vi "Set example module data API.vi"(7 "Config":T1={"Type"=enum."PTI", "Wavelength (nm)"=600.0, "Wavelength (nm)"="600 nm", "Grating, gr/mm"=2, "Grating mode"=enum."Unknown", "Spectrum mode"={"Spectrum mode?"=FALSE, "Start wavelength (nm)"=0.0, "End wavelength (nm)"=0.0, "Wavelength step (nm)"=0.0, "Wavelength array"=[], "array index"=0}, "VISA"={"delay before read (ms)"=50, "Mono 1"={"Timeout (ms)"=1000, "Resource Name"="COM1", "Baud Rate"=9600, "Data Bits"=8, "Parity"=0, "Stop Bits"=10, "Flow Control"=0}, "Mono 2"={"Timeout (ms)"=1000, "Resource Name"="COM1", "Baud Rate"=9600, "Data Bits"=8, "Parity"=0, "Stop Bits"=10, "Flow Control"=0}}} {"VISA"."Mono 2"."Flow Control" items=["1.0"=10, "1.5"=15, "2.0"=20]; "VISA"."Mono 2"."Stop Bits" items=["None", "Odd", "Even", "Mark", "Space"]; "VISA"."Mono 2"."Parity" items=["None", "Odd", "Even", "Mark", "Space"]; "VISA"."Mono 1"."Flow Control" items=["1.0"=10, "1.5"=15, "2.0"=20]; "VISA"."Mono 1"."Stop Bits" items=["None", "Odd", "Even", "Mark", "Space"]; "VISA"."Mono 1"."Parity" items=["None", "Odd", "Even", "Mark", "Space"]; "Grating, gr/mm" items=["2400", "1800", "1200", "600", "300", "150"]}, 8 "Error In":errorcluster) -> (0 "Error Out":errorcluster)   [LabVIEW 2017, in "Main controller.lvlib"]
uses:
  Main controller.lvlib
  Example Module/Controls/Params.ctl
  Monochromator/Controls/Grating.ctl
  Monochromator/Controls/VISA parameters.ctl
  CTLs/Command Data [cluster].ctl
  CTLs/Commands [enum].ctl
  Events/Events.lvlib
  Serial comms/Serial comms.lvlib
  Monochromator/Monochromator.lvlib
  Example Module/Example Module.lvlib
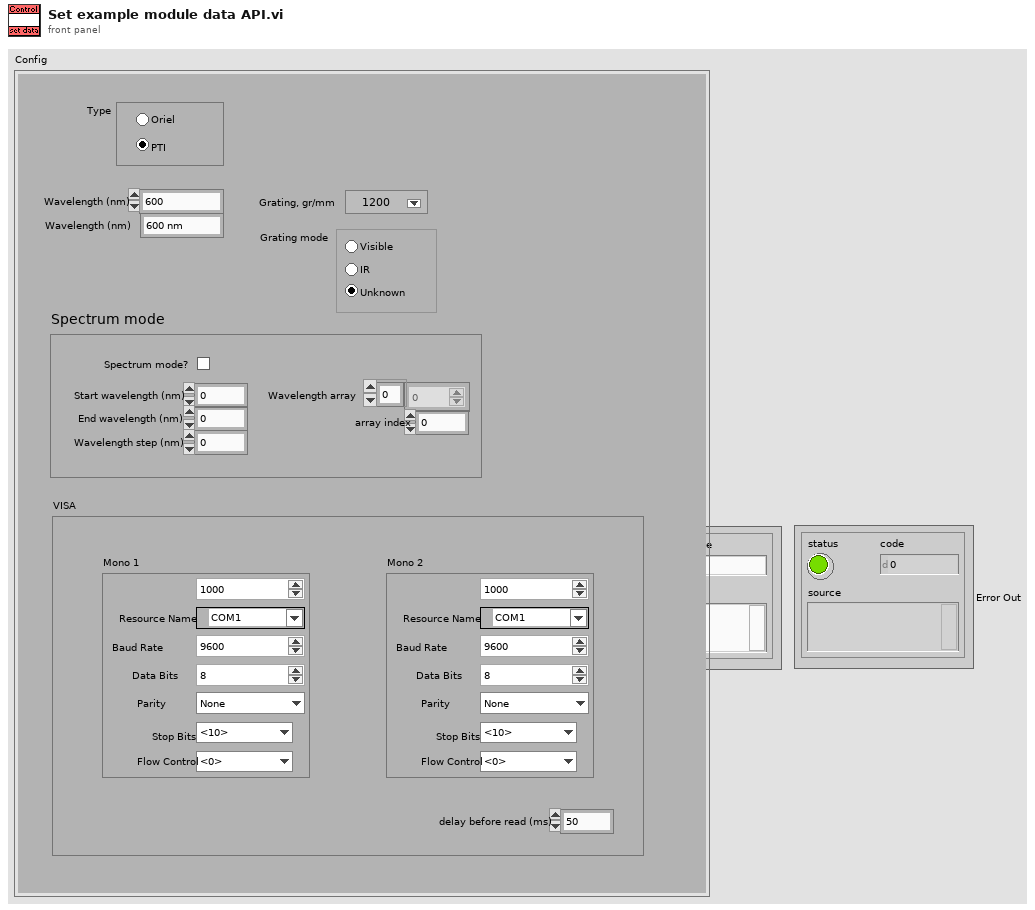
[diagram p1: front panel]
types:
  T1 = typedef "Example Module.lvlib/Params.ctl" = cluster{"Type":enum32{"Oriel", "PTI"}, "Wavelength (nm)":dbl, "Wavelength (nm)":string, "Grating, gr/mm":u16, "Grating mode":T2, "Spectrum mode":cluster{"Spectrum mode?":bool, "Start wavelength (nm)":dbl, "End wavelength (nm)":dbl, "Wavelength step (nm)":dbl, "Wavelength array":dbl[], "array index":u32}, "VISA":cluster{"delay before read (ms)":u32, "Mono 1":T3, "Mono 2":T3}}
  T2 = typedef "Monochromator.lvlib/Grating.ctl" = enum32{"Unknown", "Visible", "IR"}
  T3 = typedef "Serial comms.lvlib/VISA parameters.ctl" = cluster{"Timeout (ms)":u32, "Resource Name":refnum<visa-resource-name>, "Baud Rate":u32, "Data Bits":u16, "Parity":u16, "Stop Bits":u16, "Flow Control":u16}
  T4 = typedef "Main controller.lvlib/Command Data [cluster].ctl" = cluster{"Command":T5, "Data":variant}
  T5 = typedef "Main controller.lvlib/Commands [enum].ctl" = enum16{"Start", "Initialise Devices", "Stop", "Set DAQ data", "Set Scope data", "Set Spectrum Setup", "Spectrum Setup Complete", "Set Monochromator Setup", "Monochromator Setup Complete", "Set Monochromator data", "Set Colour Wheel Setup", "Colour Wheel Setup Complete", "Move Shutter", "Move Shutter Complete", "Collect Data", "DAQ Acquisition Complete", "Scope Acquisition Complete", "Collect Data Complete", "A-B Processing", "A-B Processing Complete", "DAQ-Scope Stitching", "DAQ-Scope Stitching Complete", "Return Shutter", "Return Shutter Complete", "Set colour wheel data", "Set all config data", "Acquire test data", "Accumulate test data", "Average test data", "All Averaging Complete", "DAQ Averaging Complete", "Scope Averaging Complete", "Finalise test data", "All Finalising Complete", "DAQ Finalising Complete", "Scope Finalising Complete", "Process test data", "End Test"}
  T6 = typedef "Events.lvlib/Refs [cluster].ctl" = cluster{"Exit":refnum<user-event>, "Controller":refnum<user-event>, "System Error":refnum<user-event>, "UI":refnum<user-event>, "Example Module":refnum<user-event>, "Shutter":refnum<user-event>, "Monochromator":refnum<user-event>, "DAQ":refnum<user-event>, "Scope":refnum<user-event>, "Processing":refnum<user-event>, "File IO":refnum<user-event>, "Colour wheel":refnum<user-event>}
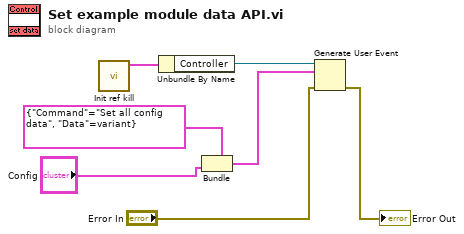
[diagram p0: block diagram]
diagram:
  n1 = call "Init ref kill.vi"() -> ("Messages"=w7:T6)  [unwired: 10 in, 1 out]
  n2 = Unbundle By Name(w7) -> ("Controller"=w6:refnum<user-event>)
  n3 = Bundle(cluster=T4 {"Command"=enum."Set all config data", "Data"=variant} ("event data"), "Data"="Config") -> (w2:T4)  [unwired: 1 in]
  n4 = Generate User Event(user event=w6, event data cluster=w2, error in="Error In") -> (error out=→"Error Out":errorcluster)  [unwired: 1 in, 1 out]
